vi "Retrieve Julian Dates.vi"(11 "Date Time (UTC)":T1) -> (2 "Julian Day":dbl, 3 "Julian Century":dbl, 5 "Timestamp (local)":timestamp)   [LabVIEW 2013, in "Solar Calculations.lvlib"]
uses:
  <vilib>/Utility/miscctls.llb/LVDateTimeRec.ctl
  Solar Calculations.lvlib
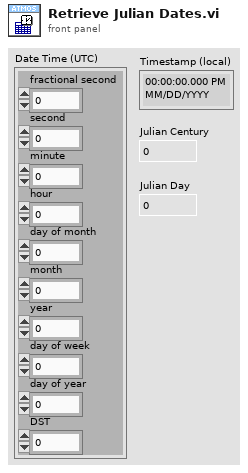
[diagram p1: front panel]
types:
  T1 = typedef "LVDateTimeRec.ctl" = cluster{"fractional second":dbl, "second":i32, "minute":i32, "hour":i32, "day of month":i32, "month":i32, "year":i32, "day of week":i32, "day of year":i32, "DST":i32}
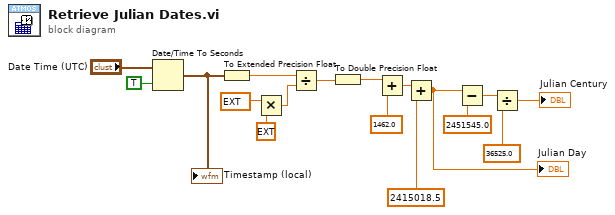
[diagram p0: block diagram]
diagram:
  n1 = Date/Time To Seconds(1:TRUE ("is UTC (F)"), 2:"Date Time (UTC)") -> (0:w5:timestamp)
  "Timestamp (local)" <- w5
  n2 = To Extended Precision Float(1:w5) -> (0:w6:ext)
  n3 = Multiply(x=ext 3600.0 ("y"), y=ext 24.0) -> (x*y=w10:ext)
  n4 = Divide(x=w6, y=w10) -> (x/y=w4:ext)
  n5 = To Double Precision Float(number=w4) -> (double precision float=w3:dbl)
  n6 = Add(x=w3, y=1462.0) -> (x+y=w11:dbl)
  n7 = Add(x=w11, y=2415018.5) -> (x+y=w13:dbl)
  "Julian Day" <- w13
  n8 = Subtract(x=w13, y=2451545.0) -> (x-y=w15:dbl)
  n9 = Divide(x=w15, y=36525.0) -> (x/y=→"Julian Century":dbl)
